vi "Archiver-Delete.vi"(8 "error in":errorcluster, 10 "files to remove":path[](array[path])) -> (0 "error out":errorcluster)   [LabVIEW 2016]
uses:
  Archiver.Action.ctl
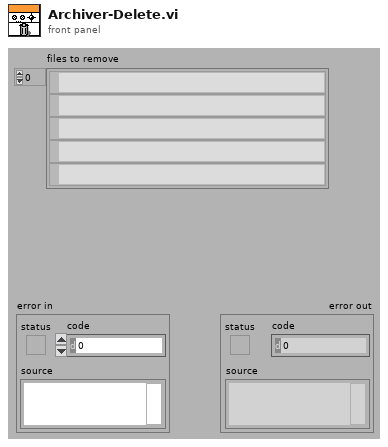
[diagram p1: front panel]
types:
  T1 = typedef "Archiver.Action.ctl" = enum32{"idle", "constructor", "destructor", "--- Archiver ---"}
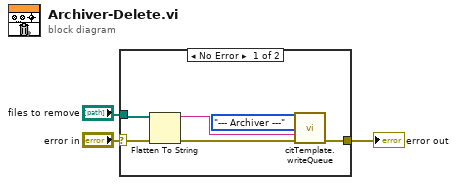
[diagram p0: block diagram]
diagram:
  n1 = case shown="No Error" "error in" {
    selector: "error in" -> [w7 w10]
    tunnel: [w9 w10] -> w2
    tunnel: "files to remove" -> [w6 _]
    frame No Error {
      n2 = Flatten To String(anything=w6, error in (no error)=w7) -> (data string=w5:string, error out=w4:errorcluster)  [unwired: 2 in, 1 out]
      n3 = call "citTemplate.writeQueue.vi"("event in (if not connected:all statemachine with data event)"=Archiver.Action."--- Archiver ---" ("Action"), "data in"=w5, "error in (no error)"=w4) -> ("error out"=w9:errorcluster)  [unwired: 12 in]
    }
    frame Error {
    }
  }
  "error out" <- w2
